vi "Does Line Intersect Vertical Edge.vi"(10 "Vertical Edge":T1, 11 "Line":T1) -> (3 "Intersects?":bool)   [LabVIEW 2021, in "Collision.lvlib"]
uses:
  Collision.lvlib
  Vector 2D/Vector 2D.lvclass
  Vector 2D/Vector 2D.lvclass/Vector 2D.ctl
  Utility/Typedef/Line.ctl
  Utility/Utility.lvlib
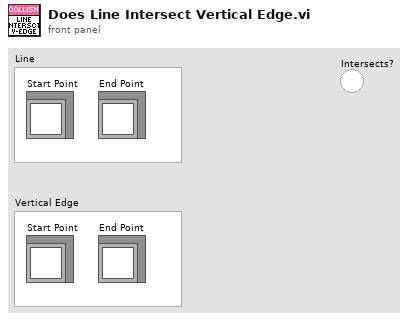
[diagram p1: front panel]
types:
  T1 = typedef "Utility.lvlib/Line.ctl" = cluster{"Start Point":refnum<class "Vector 2D.lvclass">, "End Point":refnum<class "Vector 2D.lvclass">}
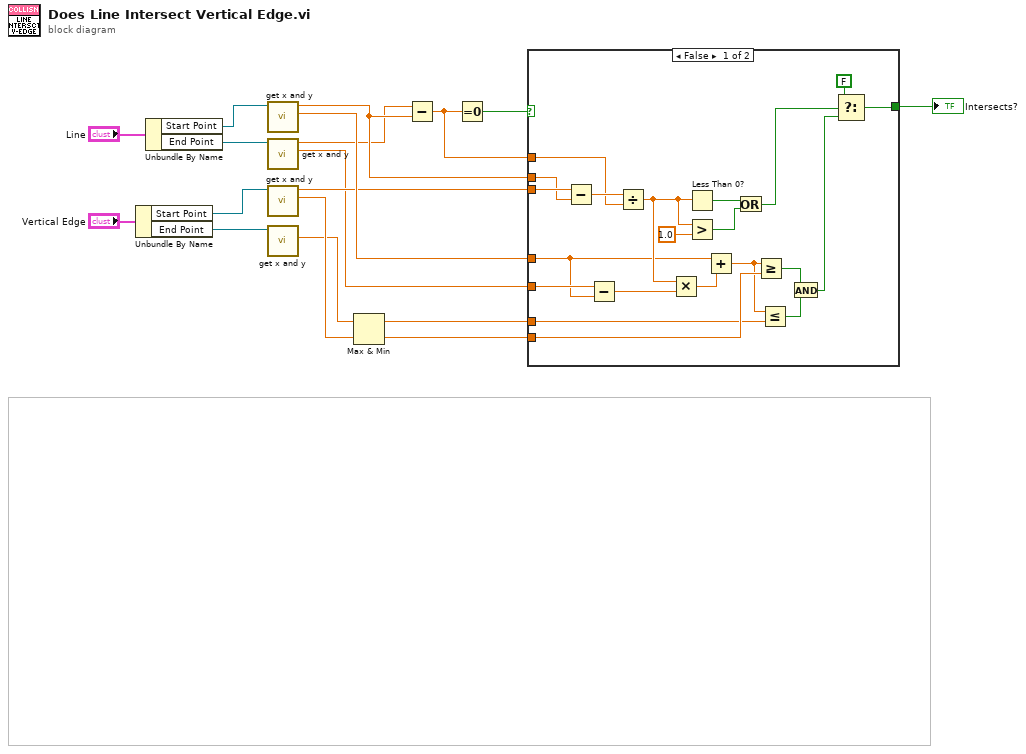
[diagram p0: block diagram]
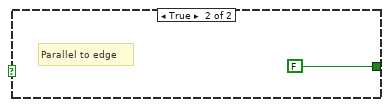
[diagram p2: hidden frame]
diagram:
  n1 = Unbundle By Name("Vertical Edge") -> ("Start Point"=w12:refnum<class "Vector 2D.lvclass">, "End Point"=w11:refnum<class "Vector 2D.lvclass">)
  n2 = Unbundle By Name("Line") -> ("Start Point"=w16:refnum<class "Vector 2D.lvclass">, "End Point"=w15:refnum<class "Vector 2D.lvclass">)
  n3 = call "get x and y.vi"("Vector 2D in"=w16) -> ("y"=w6:sgl, "x"=w7:sgl)  [unwired: 9 in]
  n4 = call "get x and y.vi"("Vector 2D in"=w15) -> ("y"=w1:sgl, "x"=w5:sgl)  [unwired: 9 in]
  n5 = call "get x and y.vi"("Vector 2D in"=w12) -> ("y"=w4:sgl, "x"=w3:sgl)  [unwired: 9 in]
  n6 = call "get x and y.vi"("Vector 2D in"=w11) -> ("y"=w2:sgl)  [unwired: 9 in, 1 out]
  n7 = Max & Min(x=w2, y=w4) -> (max(x,y)=w9:sgl, min(x,y)=w8:sgl)
  n8 = Subtract(x=w5, y=w7) -> (x-y=w10:sgl)
  n9 = Equal To 0?(x=w10) -> (x = 0?=w14:bool)
  n10 = case shown="False" w14 {
    tunnel: [w30 FALSE] -> w13
    tunnel: w3 -> [w39 _]
    tunnel: w7 -> [w38 _]
    tunnel: w10 -> [w36 _]
    tunnel: w6 -> [w26 _]
    tunnel: w1 -> [w29 _]
    tunnel: w9 -> [w22 _]
    tunnel: w8 -> [w24 _]
    frame False {
      n11 = Subtract(x=w39, y=w38) -> (x-y=w37:sgl)
      n12 = Subtract(x=w29, y=w26) -> (x-y=w28:sgl)
      n13 = Divide(x=w37, y=w36) -> (x/y=w27:sgl)
      n14 = Multiply(x=w27, y=w28) -> (x*y=w25:sgl)
      n15 = Less Than 0?(x=w27) -> (x < 0?=w35:bool)
      n16 = Greater?(x=w27, y=sgl 1.0) -> (0:w33:bool)
      n17 = Add(x=w26, y=w25) -> (x+y=w23:sgl)
      n18 = Or(x=w35, y=w33) -> (x .or. y?=w32:bool)
      n19 = Greater Or Equal?(x=w23, y=w24) -> (x >= y?=w21:bool)
      n20 = Less Or Equal?(x=w23, y=w22) -> (x <= y?=w20:bool)
      n21 = And(x=w21, y=w20) -> (x .and. y?=w19:bool)
      n22 = Select(t=FALSE, s=w32, f=w19) -> (s? t:f=w30:bool)
    }
    frame True {
      # "Parallel to edge"
    }
  }
  "Intersects?" <- w13
